vi "TwH5TranslateReturnValue.vi"(1 "TwRetVal":i32) -> (0 "return type":string)   [LabVIEW 2009]
uses:
  TwH5Dll.dll
panel:
  in  "error in (no error)":errorcluster
  out "error out":errorcluster
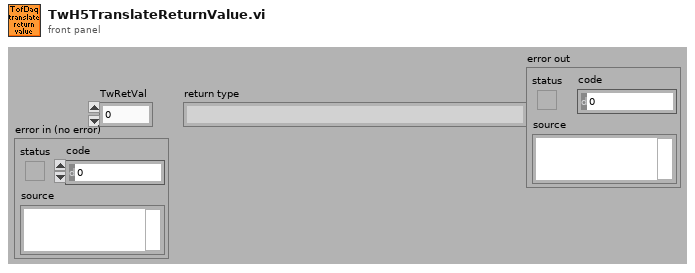
[diagram p1: front panel]
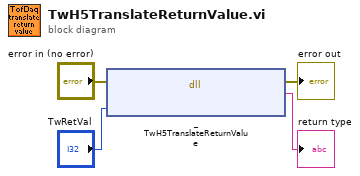
[diagram p0: block diagram]
diagram:
  n1 = dll-call lib="C:/src/85_TofDaq_current/DllWrappers/LabView/TwH5Dll/TwH5Dll.dll" fn="_TwH5TranslateReturnValue"(error in="error in (no error)", "TwRetVal"="TwRetVal") -> (error out=→"error out":errorcluster, "return type"=→"return type":string)  [unwired: 3 in, 1 out]
